vi "Enable-Disable Dynamic Shunt Cal.vi"(8 "error in":errorcluster, 10 "Dynamic shunt?":bool, 11 "Node Ptr in":T1 format="%.0x") -> (0 "error out":errorcluster, 3 "Node Ptr out":T1 format="%.0x")   [LabVIEW 2017, in "Modules.lvlib" / "9237.lvclass"]
uses:
  9237.lvclass
  <vilib>/NI Veristand/Custom Device API/Custom Device Item Ref.ctl
  C:/Users/dbuck/Documents/GitHub/Scan-Engine-Custom-Device-Classes/Source/RSI Module/RSI Module.lvclass
  9237.lvclass/9237.ctl
  <vilib>/NI Veristand/Custom Device API/Custom Device Channel.ctl
  <vilib>/NI Veristand/Custom Device API/Custom Device Channel Type.ctl
  RSI Module/Channel GUIDs.vi
  <vilib>/NI Veristand/Custom Device Tools/Custom Device Utility Library/NI VeriStand - Search for Item by GUID.vi
  <vilib>/NI Veristand/Custom Device Tools/Custom Device Utility Library/Custom Device Utility Library.lvlib
  RSI Module/RSI Module.lvclass
  <vilib>/NI Veristand/Custom Device API/Custom Device API.lvlib
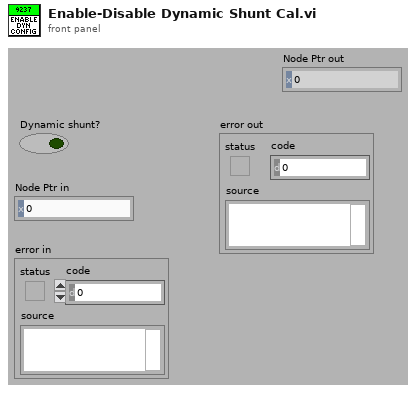
[diagram p1: front panel]
types:
  T1 = typedef "Custom Device API.lvlib/Custom Device Item Ref.ctl" = u64
  T2 = typedef "Custom Device API.lvlib/Custom Device Channel.ctl" = cluster{"Type":T3, "Units":string, "Default Value":dbl, "Faultable":bool, "Scalable":bool}
  T3 = typedef "Custom Device API.lvlib/Custom Device Channel Type.ctl" = enum16{"Input", "Output"}
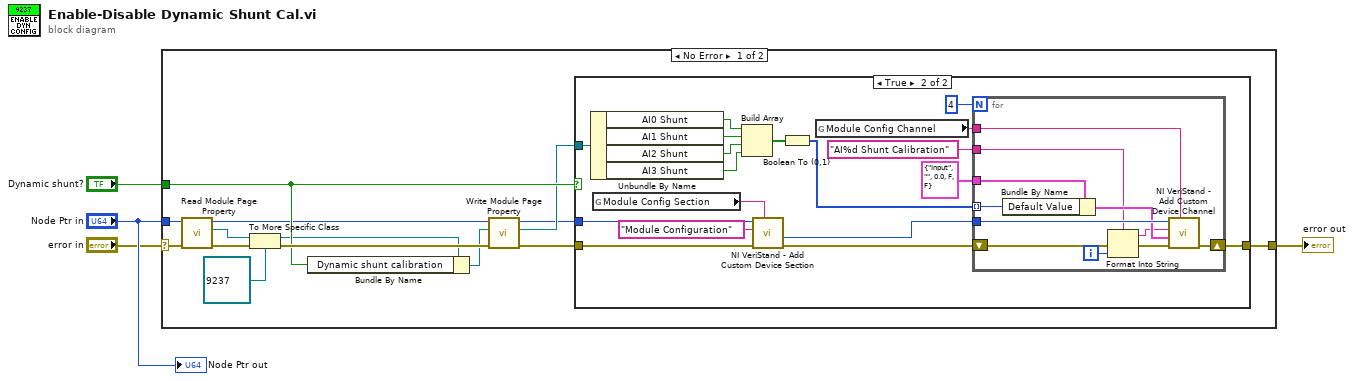
[diagram p0: block diagram]
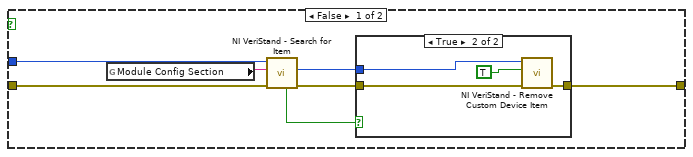
[diagram p2: hidden frame]
diagram:
  n1 = case shown="No Error" "error in" {
    selector: "error in" -> [w16 w60]
    tunnel: [w5 w60] -> w4
    tunnel: "Node Ptr in" -> [w18 _]
    tunnel: "Dynamic shunt?" -> [w12 _]
    frame No Error {
      n2 = call "Read Module Page Property.vi"("error in (no error)"=w16, "Node Ptr In"=w18) -> ("error out"=w15:errorcluster, "RSI Module"=w14:refnum<class "RSI Module.lvclass">, "Node Ptr Out"=w9:T1)  [unwired: 7 in]
      n3 = To More Specific Class(target class=refnum<class "9237.lvclass"> refnum ("9205 in"), reference=w14, error in=w15) -> (specific class reference=w11:refnum<class "9237.lvclass">, error out=w13:errorcluster)
      n4 = Bundle By Name(cluster=w11, "Dynamic shunt calibration"=w12) -> (w10:refnum<class "9237.lvclass">)
      n5 = call "Write Module Page Property.vi"("error in (no error)"=w13, "RSI Module"=w10, "Node Ptr In"=w9) -> ("error out"=w6:errorcluster, "RSI Module out"=w8:refnum<class "9237.lvclass">, "Node Ptr Out"=w7:T1)  [unwired: 6 in]
      n6 = case shown="True" w12 {
        tunnel: w7 -> [w25 w48]
        tunnel: w6 -> [w24 w47]
        tunnel: [w19 w33] -> w5
        tunnel: w8 -> [_ w32]
        frame False {
          n7 = global read "Channel GUIDs.vi" "Module Config Section"() -> (w23:string)
          n8 = call-poly <vilib>:"NI VeriStand - Search for Item.vi"("error in"=w24, "Item GUID"=w23, "Section Ref in"=w25) -> ("error out"=w21:errorcluster, "Item Ref"=w20:T1, "Found"=w22:bool)  [unwired: 5 in, 1 out]
          n9 = case shown="True" w22 {
            tunnel: w21 -> [w26 w30]
            tunnel: w20 -> [_ w29]
            tunnel: [w26 w27] -> w19
            frame False {
            }
            frame True {
              n10 = call <vilib>:"NI VeriStand - Remove Custom Device Item.vi"("error in (no error)"=w30, "Force Delete (F)"=TRUE, "Item Ref in"=w29) -> ("error out"=w27:errorcluster)  [unwired: 7 in, 1 out]
            }
          }
        }
        frame True {
          n11 = Unbundle By Name(w32) -> ("AI0 Shunt"=w41:bool, "AI1 Shunt"=w40:bool, "AI2 Shunt"=w39:bool, "AI3 Shunt"=w38:bool)
          n12 = global read "Channel GUIDs.vi" "Module Config Section"() -> (w46:string)
          n13 = Build Array(w41, w40, w39, w38) -> (w36:bool[])
          n14 = call <vilib>:"NI VeriStand - Add Custom Device Section.vi"("GUID (Default Section)"=w46, "error in (no error)"=w47, "Section Name"="Module Configuration", "Parent Ref in"=w48) -> ("error out"=w43:errorcluster, "Section Ptr"=w31:T1)  [unwired: 4 in, 2 out]
          n15 = Boolean To (0,1)(Boolean=w36) -> (0, 1=w35:i16[])
          n16 = global read "Channel GUIDs.vi" "Module Config Channel"() -> (w42:string)
          n17 = for {
            N: 4 -> [_]
            tunnel: w31 -> [w59]
            shift-right: [w58] -> w33
            shift-left: w43 -> [w51]
            tunnel: w42 -> [w57]
            tunnel: T2 {"Type"=enum."Input", "Units"="", "Default Value"=0.0, "Faultable"=FALSE, "Scalable"=FALSE} ("Channel") -> [w56]
            tunnel: w35 -> [w55] mode=indexing
            tunnel: "AI%d Shunt Calibration" ("Channel Name") -> [w53]
            i -> [w52]
            n18 = Bundle By Name(cluster=w56, "Default Value"=w55) -> (w54:T2)
            n19 = Format Into String(format string=w53, error in=w51, w52) -> (resulting string=w49:string, error out=w50:errorcluster)  [unwired: 1 in]
            n20 = call <vilib>:"NI VeriStand - Add Custom Device Channel.vi"("GUID (Default Channel)"=w57, "error in (no error)"=w50, "Channel"=w54, "Channel Name"=w49, "Parent Ref in"=w59) -> ("error out"=w58:errorcluster)  [unwired: 3 in, 3 out]
          }
        }
      }
    }
    frame Error {
    }
  }
  "error out" <- w4
  "Node Ptr out" <- "Node Ptr in"
